vi "Exactly Matching String Inputs.vi"(7 "Expected Number of Calls":u32, 8 "error in (no error)":errorcluster, 11 "Mock in":refnum<class "LMock Mock.lvclass">) -> (0 "error out":errorcluster, 3 "Mock out":refnum<class "LMock Mock.lvclass">)   [LabVIEW 2020, in "Deprecated Exactly.lvlib"]
doc: "This VI has been deprecated and will be removed in a future version of LMock. \nPlease use LMock Exactly.vi instead."
uses:
  Deprecated Exactly.lvlib
  Framework/Mock/LMock Mock.lvclass
  Comparators/Matching String Input Comparator/Matching String Input Comparator.lvclass
  C:/git/astemes-lmock/source/Core/Comparator/Comparator.lvclass
  Exactly.lvclass
  C:/git/astemes-lmock/source/Core/Expectation/Expectation.lvclass
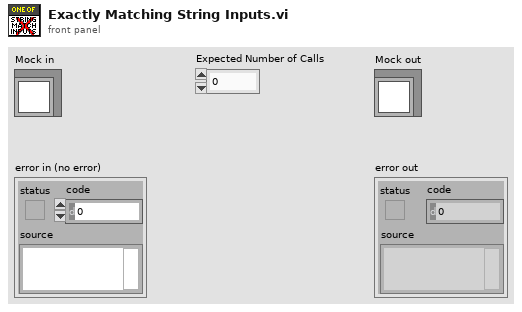
[diagram p1: front panel]
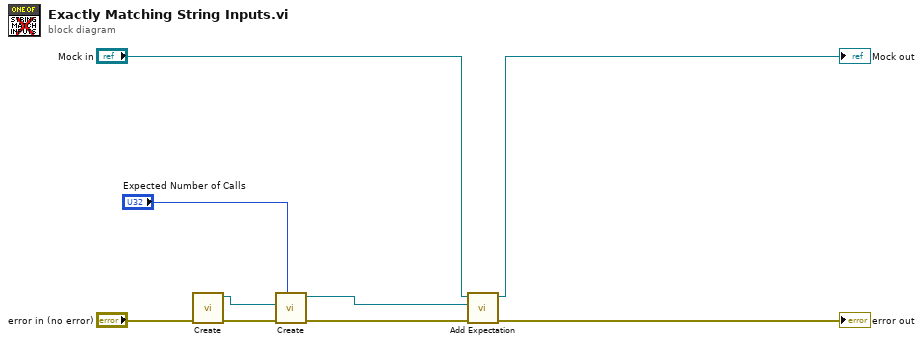
[diagram p0: block diagram]
diagram:
  n1 = call "Create.vi"("error in (no error)"="error in (no error)") -> ("error out"=w2:errorcluster, "String Argument Matching Comparator"=w4:refnum<class "Matching String Input Comparator.lvclass">)  [unwired: 9 in]
  n2 = call "Create.vi"("Expected Number of Calls"="Expected Number of Calls", "error in (no error)"=w2, "Comparator"=w4) -> ("error out"=w6:errorcluster, "Exactly Out"=w5:refnum<class "Exactly.lvclass">)  [unwired: 7 in]
  n3 = call-dynamic "Add Expectation.vi"("error in (no error)"=w6, "Expectations"=w5, "Mock in"="Mock in") -> ("error out"=→"error out":errorcluster, "Mock out"=→"Mock out":refnum<class "LMock Mock.lvclass">)  [unwired: 7 in]
